vi "PH_Beamline.Calc Experiment LB State.vi"(0 "i ref in":refnum<vi>, 5 "error in (no error)":errorcluster) -> (14 "i ref out":refnum<vi>, 19 "error out":errorcluster)   [LabVIEW 2014, in "PH_Beamline.lvlib"]
doc: "This VI calculates the experiment laserbay state of the Beamline."
uses:
  PH_Beamline.lvlib
  PH_Basics/PH_SystemInformation/PH_SystemInformationEnabling State.ctl
  PH_Basics/PH_Common/PH_Common.lvlib
  PH_Basics/PH_SystemInformation/PH_SystemInformation.lvlib
  PH_BL-Master/PH_BL-Master.lvlib
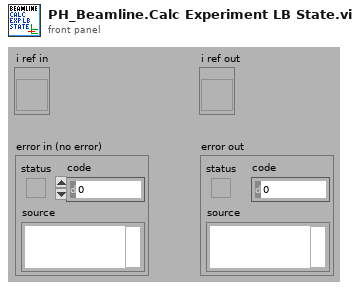
[diagram p1: front panel]
types:
  T1 = typedef "PH_Beamline.lvlib/PH_Beamline.i attribute.ctl" = cluster{"GUI Refs":cluster{"PA ok":refnum<vi>, "MA ok":refnum<vi>, "fs FE ok":refnum<vi>, "ns FE ok":refnum<vi>, "PA ED ok":refnum<vi>, "MAS ok":refnum<vi>, "Booster ok":refnum<vi>, "Mirrortower ok":refnum<vi>, "In.-Box ok":refnum<vi>, "Compressor ok":refnum<vi>, "Experiment LB ok":refnum<vi>, "Experiment LL ok":refnum<vi>, "PHELIX_Beckhoff_Watchdog":refnum<vi>, "Shutters closed":refnum<vi>, "uOPA ok":refnum<vi>, "Vacuum no shotcond Comp LB":refnum<vi>}, "Refs BL MA":refnum<vi>[], "Refs BL MA-IB":refnum<vi>[], "Refs BL fs":refnum<vi>[], "Refs BL PA ED":refnum<vi>[], "Refs BL MAS":refnum<vi>[], "Refs BL Boo":refnum<vi>[], "Refs BL ns":refnum<vi>[], "Refs BL Mirrortower":refnum<vi>[], "Refs BL Compressor":refnum<vi>[], "Refs BL Exp LB":refnum<vi>[], "Radiation Safety":cluster{"Exp Laserbay":cluster{"Ref Op Mode":refnum<vi>, "Ref Laserbay evacuated":refnum<vi>, "Tagname LB evacuated":string, "Shot Mode":T2, "Laserbay evacuated?":i32, "Tagname HV room locked":string, "HV room locked?":i32, "Ref HV room locked":refnum<vi>, "Tagname bridged?":string, "Ref Bridge":refnum<vi>, "I<1E18W/cm²":bool}, "Exp Laserlab":cluster{"Ref Op Mode":refnum<vi>, "Ref Laserlab evacuated":refnum<vi>, "Tagname LL evacuated":string, "Shot Mode":T2, "Laserlab evacuated?":i32, "Tagname bridged?":string, "Ref Bridge":refnum<vi>, "I<1E18W/cm²":bool}}, "Refs BL LL":refnum<vi>[], "PP Igni Heating GUI Refs":refnum<vi>[], "PP Igni Heating Tagnames ":string[], "Refs BL PA":cluster{"undelayed Line before Shutter":refnum<vi>[], "undelayed Line after Shutter":refnum<vi>[], "before Bypass":refnum<vi>[], "delayed Line before Shutter":refnum<vi>[], "delayed Line after Shutter":refnum<vi>[], "before Shutter Input":refnum<vi>[], "after Shutter Input":refnum<vi>[], "Bypass":refnum<vi>[], "before Shutter Exit":refnum<vi>[], "after Shutter Exit":refnum<vi>[], "to MA":refnum<vi>[], "to Lab":refnum<vi>[]}, "BL":cluster{"YLF_BL_Status":i32, "fs_BL_Status":i32, "fs_YLF_BL_Status":i32, "ns_BL_Status":i32, "PA_Input_BL_Status":i32, "PA_UnDelay_BL_Status":i32, "PA_Delay_BL_Status":i32, "PA_BL_Status":i32, "PA_Bypass_BL_Status":i32, "PA_Exit_BL_Status":i32, "PA_LL_BL_Status":i32, "LL_BL_Status":i32, "PA_MA_BL_Status":i32, "MA_Exit_BL_Status":i32, "MA_Z6_BL_Status":i32, "Z6_BL_Status":i32, "MA_LB_BL_Status":i32, "LB_TB2_BL_Status":i32, "PA_before_Bypass_BL_Status":i32, "LB_TB3_BL_Status":i32}, "State Subsystems":cluster{"PA":bool, "MA":bool, "ns FE":bool, "fs FE":bool, "PA ED":bool, "In.-Box":bool, "MAS":bool, "Booster":bool, "Mirrortower":bool, "Compressor":bool, "Experiment LB":bool, "Experiment LL":bool, "uOPA":bool}, "Status Subscriber Information":T3, "Refs BL uOPA":refnum<vi>[], "PA_Input_2_Beam_6PWpGUI not linked?":bool, "PA_Input_Delay_6PGUI not linked?":bool, "Settings":T6}
  T2 = typedef "PH_Beamline.lvlib/PH_Beamline.Operation Mode.ctl" = i32
  T3 = typedef "PH_Beamline.lvlib/PH_Beamline.Status Subscriber Information.ctl" = cluster{"fs Swich YLF":T4, "fs Exit Shutter":T4, "ns Exit Shutter":T4, "PA Input Shutter":T4, "PA PC WP":T4, "PA PC WP 2":T4, "PA Bypass In":T4, "PA Bypass Out":T4, "PA CH 1":T4, "PA delayed":T4, "PA non delayed":T4, "PA Exit Shutter":T4, "PA Switch Lab":T4, "PA Bridge CH Input MA":T4, "MA Diffusor IB":T4, "MA IB Ready":T4, "MA CH 1":T4, "MA CH 2":T4, "MA CH 3":T4, "MA CH 4":T4, "MA Shutter Align Cam":T4, "MA Position MM5":T4, "Calorimeter Switch":T4, "BL Z6 CH 9":T4, "BL Z6 Beamdump":T4, "BL Z6 Shutter":T4, "COS Sensitivity Switch":T4, "Exp LB Shutter":T4, "Exp LB TB 2":T4, "Exp LB TB 3":T4, "PA LL Input CH":T4, "PA LL Output CH":T4, "LL Comp Input Shutter":T4, "LL Comp Output Shutter":T4, "LL Comp FF Shutter":T4, "Exp LL Shutter":T4, "MA IM In IB":T4, "MA IM Out IB":T4, "MA DB In IB":T4, "MA DB Out IB":T4, "Exp LB Shutter Interlock":T4, "Exp LL Shutter Interlock":T4, "MM1 Force Sensor":T4}
  T4 = typedef "PH_BL-Master.lvlib/PH_BL-Master.Status Subscriber Information.ctl" = cluster{"Index of element":i32, "Attributeset":T5}
  T5 = typedef "PH_BL-Master.lvlib/PH_BL-Master.Attribute Set.ctl" = enum16{"Boolean Status Service Subscriber", "Picture Status Service Subscriber"}
  T6 = typedef "PH_Beamline_Chief.lvlib/PH_Beamline_Chief.Settings.ctl" = cluster{"PA Doublepass Mode":bool, "Compressor Vaccuum LB not relevant":bool, "Windowshutter TB2 not relevant":bool, "Windowshutter TB3 not relevant":bool}
  T7 = enum16{"Laser", "PreAmp", "MainAmp", "Exp 1", "Exp 2", "Exp 3", "Exp 4"}[]
  T8 = typedef "PH_SystemInformation.lvlib/PH_SystemInformationEnabling State.ctl" = i32
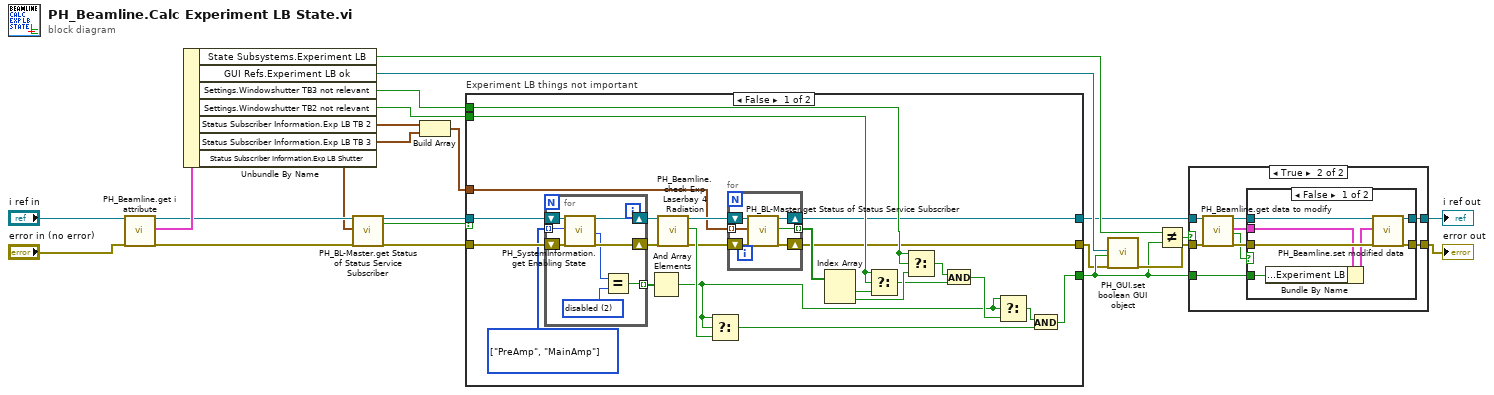
[diagram p0: block diagram]
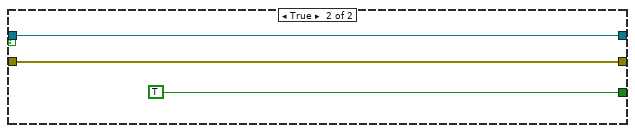
[diagram p4: hidden frame]
diagram:
  n1 = call "PH_Beamline.get i attribute.vi"("i ref in"="i ref in", "error in (no error)"="error in (no error)") -> ("i ref out"=w10:refnum<vi>, "i attribute"=w20:T1, "error out"=w9:errorcluster)  [unwired: 15 in]
  n2 = Unbundle By Name(w20) -> ("State Subsystems.Experiment LB"=w17:bool, "GUI Refs.Experiment LB ok"=w23:refnum<vi>, "Settings.Windowshutter TB3 not relevant"=w1:bool, "Settings.Windowshutter TB2 not relevant"=w2:bool, "Status Subscriber Information.Exp LB TB 2"=w6:T4, "Status Subscriber Information.Exp LB TB 3"=w5:T4, "Status Subscriber Information.Exp LB Shutter"=w4:T4)
  n3 = call "PH_BL-Master.get Status of Status Service Subscriber.vi"("i ref in"=w10, "Wanted Status Subscriber Information"=w4, "error in (no error)"=w9) -> ("i ref out"=w21:refnum<vi>, "off/false/out?"=w19:bool, "error out"=w22:errorcluster)  [unwired: 11 in, 3 out]
  n4 = Build Array(w6, w5) -> (w3:T4[])
  n5 = case "Experiment LB things not important" shown="False" w19 {
    tunnel: w21 -> [w47 w64]
    tunnel: [w25 w64] -> w8
    tunnel: w22 -> [w45 w63]
    tunnel: [w24 w63] -> w7
    tunnel: [w38 TRUE] -> w13
    tunnel: w3 -> [w28 _]
    tunnel: w2 -> [w26 _]
    tunnel: w1 -> [w27 _]
    frame False {
      w43 = T7 [enum."PreAmp", enum."MainAmp"] items=["Laser", "PreAmp", "MainAmp", "Exp 1", "Exp 2", "Exp 3", "Exp 4"]
      n6 = for {
        shift-right: [w60] -> w46
        shift-left: w47 -> [w61]
        shift-right: [w58] -> w44
        shift-left: w45 -> [w59]
        tunnel: w43 -> [w57] mode=indexing
        tunnel: [w54] -> w42 mode=indexing
        w55 = T8 2 items=["no info", "not disabled", "disabled"] ("y")
        n7 = call "PH_SystemInformation.get Enabling State.vi"("i ref in"=w61, "Wanted State"=w57, "error in (no error)"=w59) -> ("i ref out"=w60:refnum<vi>, "Enabling State"=w56:T8, "error out"=w58:errorcluster)  [unwired: 14 in]
        n8 = Equal?(x=w56, y=w55) -> (x = y?=w54:bool)
      }
      n9 = And Array Elements(Boolean array=w42) -> (logical AND=w29:bool)
      n10 = call "PH_Beamline.check Exp Laserbay 4 Radiation.vi"("i ref in"=w46, "error in"=w44) -> ("i ref out"=w39:refnum<vi>, "Laserbay save concerning Radiation"=w41:bool, "error out"=w40:errorcluster)  [unwired: 15 in]
      n11 = Select(t=w29, s=w29, f=w41) -> (s? t:f=w34:bool)
      n12 = for {
        tunnel: [w49] -> w37 mode=indexing
        shift-right: [w50] -> w25
        shift-left: w39 -> [w51]
        shift-right: [w52] -> w24
        shift-left: w40 -> [w53]
        tunnel: w28 -> [w48] mode=indexing
        n13 = call "PH_BL-Master.get Status of Status Service Subscriber.vi"("i ref in"=w51, "Wanted Status Subscriber Information"=w48, "error in (no error)"=w53) -> ("i ref out"=w50:refnum<vi>, "on/true/in?"=w49:bool, "error out"=w52:errorcluster)  [unwired: 11 in, 3 out]
      }
      n14 = Index Array(array=w37) -> (element #1=w36:bool, element #2=w35:bool)  [unwired: 2 in]
      n15 = Select(t=w26, s=w26, f=w36) -> (s? t:f=w32:bool)
      n16 = Select(t=w27, s=w27, f=w35) -> (s? t:f=w33:bool)
      n17 = And(x=w33, y=w32) -> (x .and. y?=w31:bool)
      n18 = Select(t=w29, s=w29, f=w31) -> (s? t:f=w30:bool)
      n19 = And(x=w30, y=w34) -> (x .and. y?=w38:bool)
    }
    frame True {
    }
  }
  n20 = call "PH_GUI.set boolean GUI object.vi"("Boolean Knob GUI Ref"=w23, "Value"=w13, "error in (no error)"=w7) -> ("error out"=w15:errorcluster)  [unwired: 16 in]
  n21 = Not Equal?(x=w17, y=w13) -> (x != y?=w18:bool)
  n22 = case shown="True" w18 {
    tunnel: [w66 w71] -> w16
    tunnel: [w65 w70] -> w14
    tunnel: w13 -> [_ w69]
    tunnel: w15 -> [w65 w68]
    tunnel: w8 -> [w66 w67]
    frame False {
    }
    frame True {
      n23 = call "PH_Beamline.get data to modify.vi"("i ref in"=w67, "error in (no error)"=w68) -> ("i ref out"=w74:refnum<vi>, "i attribute"=w72:T1, "timed out"=w73:bool, "error out"=w75:errorcluster)  [unwired: 14 in]
      n24 = case shown="False" w73 {
        tunnel: w75 -> [w82 w83]
        tunnel: w74 -> [w81 w84]
        tunnel: [w80 w83] -> w70
        tunnel: [w79 w84] -> w71
        tunnel: w72 -> [w78 _]
        tunnel: w69 -> [w76 _]
        frame False {
          n25 = Bundle By Name(cluster=w78, "State Subsystems.Experiment LB"=w76) -> (w77:T1)
          n26 = call "PH_Beamline.set modified data.vi"("i ref in"=w81, "i attribute"=w77, "error in (no error)"=w82) -> ("i ref out"=w79:refnum<vi>, "error out"=w80:errorcluster)  [unwired: 15 in]
        }
        frame True {
        }
      }
    }
  }
  "i ref out" <- w16
  "error out" <- w14
